vi "circularInstance.vi"(1 "data":u32[](array[numeric]), 2 "max-size":i16, 3 "element":u32) -> (0 "dataout":u32[](array[numeric]))   [LabVIEW 2013]
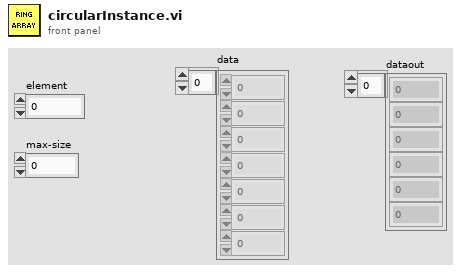
[diagram p1: front panel]
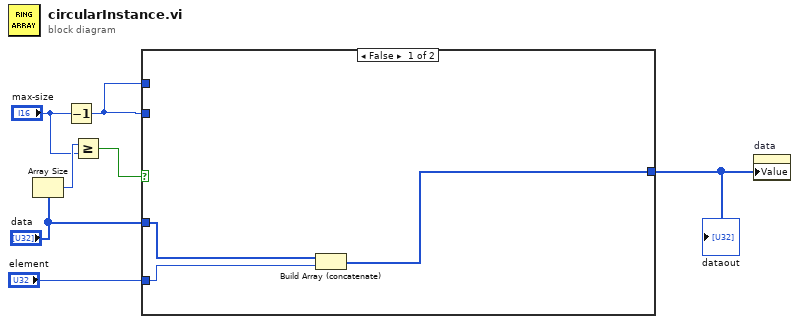
[diagram p0: block diagram]
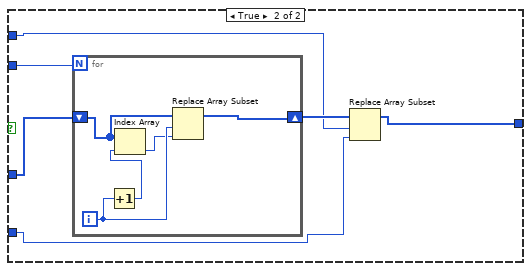
[diagram p2: hidden frame]
diagram:
  n1 = Array Size(array="data") -> (size(s)=w5:i32)
  n2 = Decrement(x="max-size") -> (x-1=w2:i16)
  n3 = Greater Or Equal?(x=w5, y="max-size") -> (x >= y?=w4:bool)
  n4 = case shown="False" w4 {
    tunnel: "data" -> [w9 w15]
    tunnel: "element" -> [w10 w13]
    tunnel: w2 -> [_ w16]
    tunnel: w2 -> [_ w12]
    tunnel: [w8 w11] -> w1
    frame False {
      n5 = Build Array (concatenate)(w9, w10) -> (w8:u32[])
    }
    frame True {
      n6 = for {
        N: w16 -> [_]
        shift-right: [w17] -> w14
        shift-left: w15 -> [w18]
        i -> [w21]
        n7 = Increment(x=w21) -> (x+1=w20:i32)
        n8 = Index Array(array=w18, index=w20) -> (element=w19:u32)
        n9 = Replace Array Subset(array=w18, new element=w19, index=w21) -> (w17:u32[])
      }
      n10 = Replace Array Subset(array=w14, new element=w13, index=w12) -> (w11:u32[])
    }
  }
  "dataout" <- w1
  n11 = property on="data" class="Arr (strict)"("Value"=w1) -> ()  [unwired: 2 in, 2 out]
